vi "Load.vi"(8 "error in (no error)":errorcluster, 11 "Serialized Configuration":string) -> (0 "error out":errorcluster, 3 "RandomNumberGenerator out":refnum<class "RandomNumberGenerator.lvclass">)   [LabVIEW 2020, in "RandomNumberGenerator.lvlib" / "RandomNumberGenerator.lvclass"]
doc: "<b>Load</b>\nThis method is called to load the configuration data into the plugin class data."
uses:
  RandomNumberGenerator.lvclass
  C:/Program Files/National Instruments/LabVIEW 2020/vi.lib/FlexLogger/SDK/PluginSDK.lvlibp/PEFClasses/SDK/Processing Element/Processing Element.lvclass
  <vilib>/FlexLogger/SDK/PluginSDK.lvlibp/PEFClasses/SDK/Processing Element/Read Parameters Property.vi
  <vilib>/FlexLogger/SDK/PluginSDK.lvlibp/PEFClasses/SDK/Parameters/Set Parameter.vi
  <vilib>/FlexLogger/SDK/PluginSDK.lvlibp/PEFClasses/SDK/Parameters/SetParameter(String).vi
  <vilib>/FlexLogger/SDK/PluginSDK.lvlibp/PEFClasses/SDK/Processing Element/Write Parameters Property.vi
  <vilib>/FlexLogger/SDK/PluginSDK.lvlibp/PEFClasses/SDK/Parameters/Parameters.lvclass
  RandomNumberGenerator.lvclass/RandomNumberGenerator.ctl
panel:
  # "#via_ignore"
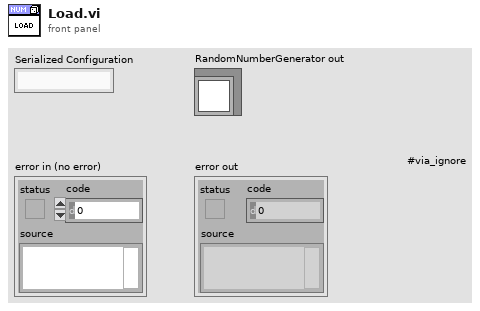
[diagram p1: front panel]
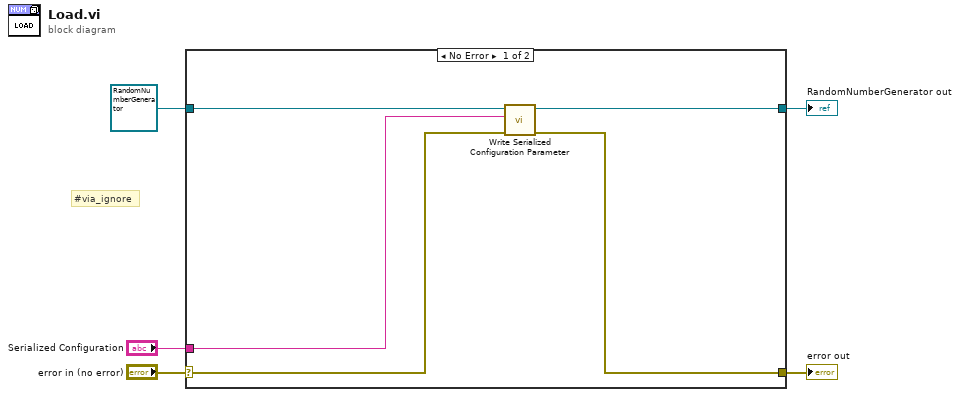
[diagram p0: block diagram]
diagram:
  # "#via_ignore"
  n1 = case shown="No Error" "error in (no error)" {
    selector: "error in (no error)" -> [w7 w12]
    tunnel: [w8 w12] -> w4
    tunnel: [w9 w11] -> w2
    tunnel: refnum<class "RandomNumberGenerator.lvclass"> refnum ("ADAS PE Template in") -> [w10 w11]
    tunnel: "Serialized Configuration" -> [w6 _]
    frame No Error {
      n2 = call "Write Serialized Configuration Parameter.vi"("error in (no error)"=w7, "Serialized Configuration"=w6, "RandomNumberGenerator in"=w10) -> ("error out"=w8:errorcluster, "RandomNumberGenerator out"=w9:refnum<class "RandomNumberGenerator.lvclass">)  [unwired: 7 in]
    }
    frame Error {
    }
  }
  "error out" <- w4
  "RandomNumberGenerator out" <- w2
